vi "Set Verbose Linker Errors.vi"(8 "error in (no error)":errorcluster, 10 "Verbose Linker Errors? (true)":bool=TRUE, 11 "PPL in":refnum<class "NI_AB_API_DPPL.lvclass">) -> (0 "error out":errorcluster, 3 "PPL out":refnum<class "NI_AB_API_DPPL.lvclass">)   [LabVIEW 2020, in "NI_AB_API_DPPL.lvclass"]
uses:
  <vilib>/AppBuilder/AB_API/DPPL/NI_AB_API_DPPL.lvclass
  <vilib>/AppBuilder/AB_API/PPL/NI_AB_API_PPL.lvclass
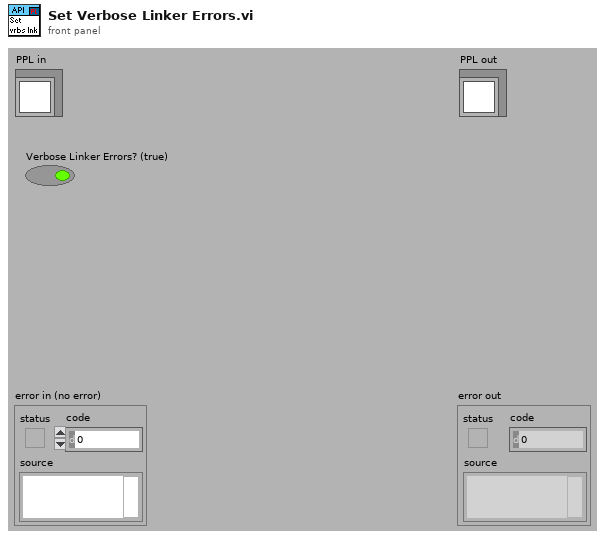
[diagram p1: front panel]
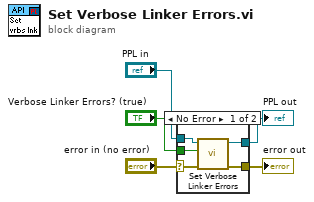
[diagram p0: block diagram]
diagram:
  n1 = case shown="No Error" "error in (no error)" {
    selector: "error in (no error)" -> [w7 w12]
    tunnel: [w8 w12] -> w4
    tunnel: [w9 w11] -> w2
    tunnel: "PPL in" -> [w10 w11]
    tunnel: "Verbose Linker Errors? (true)" -> [w6 _]
    frame No Error {
      n2 = call-parent "Set Verbose Linker Errors.vi"("error in (no error)"=w7, "Verbose Linker Errors? (true)"=w6, "PPL in"=w10) -> ("error out"=w8:errorcluster, "PPL out"=w9:refnum<class "NI_AB_API_DPPL.lvclass">)  [unwired: 7 in]
    }
    frame Error {
    }
  }
  "error out" <- w4
  "PPL out" <- w2
